vi "FRAS Construction tab X.vi"(5 "Largeur cote":i32, 9 "Tableau":i32[](array[numeric])) -> (8 "Tableau 2":i32[](array[numeric]))   [LabVIEW 2020]
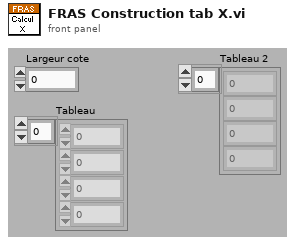
[diagram p1: front panel]
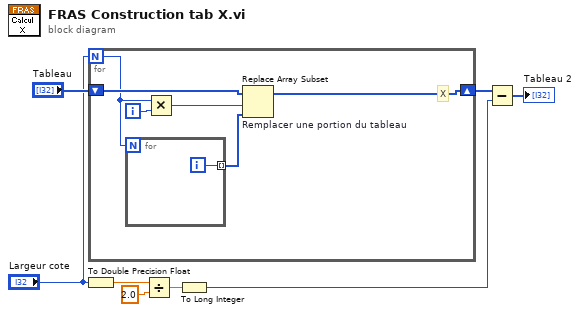
[diagram p0: block diagram]
diagram:
  n1 = To Double Precision Float(number="Largeur cote") -> (double precision float=w1:dbl)
  n2 = for {
    N: "Largeur cote" -> [w9]
    shift-right: [w13] -> w6
    shift-left: "Tableau" -> [w12]
    i -> [w14]
    # "X"
    n3 = for {
      N: w9 -> [_]
      tunnel: [w15] -> w10 mode=indexing
      i -> [w15]
    }
    n4 = Multiply(x=w9, y=w14) -> (x*y=w11:i32)
    n5 = Replace Array Subset "Remplacer une portion du tableau"(array=w12, new element=w10, index=w11) -> (w13:i32[])
  }
  n6 = Divide(x=w1, y=2.0) -> (x/y=w5:dbl)
  n7 = To Long Integer(number=w5) -> (32bit integer=w2:i32)
  n8 = Subtract(x=w6, y=w2) -> (x-y=→"Tableau 2":i32[])
